vi "Page_Source_Settings_Update_Display.vi"(6 "AB_Build in":refnum<class "AB_Build.lvclass">, 8 "error in (no error)":errorcluster, 9 "ctlReferences":T3, 10 "supportedFunctions":T2, 11 "AB_Source in":refnum<class "AB_Source.lvclass">) -> (0 "error out":errorcluster, 2 "parentApplies":T1, 3 "AB_Source out":refnum<class "AB_Source.lvclass">)   [LabVIEW 2020, in "AB_Source.lvclass"]
uses:
  <vilib>/AppBuilder/AB_Classes/Source/AB_Source.lvclass
  <resource>/Framework/Providers/Builds/AppBuilder/AB_UI_Page_Source_Settings_References.ctl
  <resource>/Framework/Providers/Builds/AppBuilder/AB_UI_Page_Source_Settings_supportedFunctions.ctl
  <vilib>/AppBuilder/AB_Parent_Applies.ctl
  <vilib>/AppBuilder/AB_Classes/Build/AB_Build.lvclass
  <vilib>/AppBuilder/AB_Classes/Source/AB_Source.lvclass/AB_Source.ctl
  <vilib>/AppBuilder/AB_Source_Inclusion.ctl
  <vilib>/AppBuilder/AB_Source_Property_Type.ctl
  <resource>/Framework/Providers/Common/provcom_StringGlobals.vi
  <vilib>/AppBuilder/AB_Classes/Destination/AB_Destination.lvclass
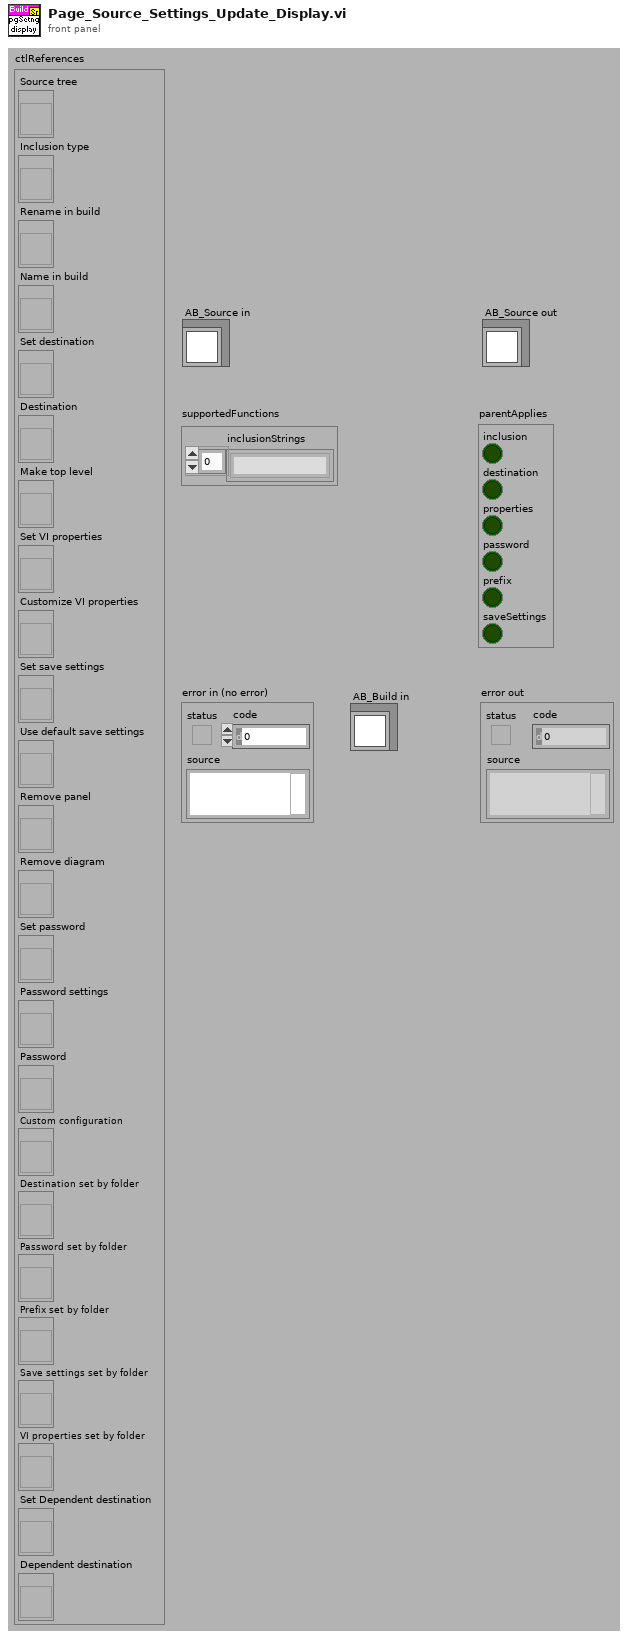
[diagram p1: front panel]
types:
  T1 = typedef "AB_Parent_Applies.ctl" = cluster{"inclusion":bool, "destination":bool, "properties":bool, "password":bool, "prefix":bool, "saveSettings":bool}
  T2 = typedef "AB_UI_Page_Source_Settings_supportedFunctions.ctl" = cluster{"inclusionStrings":string[]}
  T3 = typedef "AB_UI_Page_Source_Settings_References.ctl" = cluster{"Source tree":refnum<vi>, "Inclusion type":refnum<vi>, "Rename in build":refnum<vi>, "Name in build":refnum<vi>, "Set destination":refnum<vi>, "Destination":refnum<vi>, "Make top level":refnum<vi>, "Set VI properties":refnum<vi>, "Customize VI properties":refnum<vi>, "Set save settings":refnum<vi>, "Use default save settings":refnum<vi>, "Remove panel":refnum<vi>, "Remove diagram":refnum<vi>, "Set password":refnum<vi>, "Password settings":refnum<vi>, "Password":refnum<vi>, "Custom configuration":refnum<vi>, "Destination set by folder":refnum<vi>, "Password set by folder":refnum<vi>, "Prefix set by folder":refnum<vi>, "Save settings set by folder":refnum<vi>, "VI properties set by folder":refnum<vi>, "Set Dependent destination":refnum<vi>, "Dependent destination":refnum<vi>}
  T4 = typedef "AB_Source_Inclusion.ctl" = enum16{"IncludeIfReferenced", "Include", "Exclude", "TopLevel"}
  T5 = typedef "AB_Source_Property_Type.ctl" = enum16{"Remove block diagram", "Remove front panel", "Password", "Window has title bar", "Show menu bar", "Show vertical scroll bar", "Show horizontal scroll bar", "Show toolbar", "Show Abort button", "Show fp when called", "Window behavior", "Allow user to close window", "Window run-time position", "Run when opened", "Allow debugging", "Auto error handling", "Generate guard code", "Use stack variables", "Expression folding", "Integer only", "Inline subVI"}
  T6 = enum32{"No password change", "Remove password", "Apply new password"}
  T7 = typedef "AB_Source_Properties.ctl" = cluster{"sourcePropertyType":T5, "value":variant}
  T8 = typedef "AB_Build.ctl" = cluster{"buildSpecName":string, "buildSpecDescription":string, "destinations":refnum<class "AB_Destination.lvclass">[], "exclusionOption":T9, "defaultLanguage":string, "supportedLanguages":string[], "excludedDirectories":path[], "buildContext":refnum<vi>, "buildObject":T10, "preview":bool, "programatic":bool, "progressBarEvents":T11, "userLog_Path":path, "preActionID":string, "preAction_Path":path, "postActionID":string, "postAction_Path":path, "eng_checkForBrokenVIs?":bool, "eng_verboseLinkerErrors?":bool, "localDest_Path":path, "targetDest_Path":path, "removeVIObject":u16, "cache":refnum<class "PreviewCache.lvclass">, "use cache":bool, "previewCache_ID":string, "buildCache_ID":string, "eng_TempLocalDest_Path":path, "eng_collectDependencies?":bool, "versionInfo":cluster{"buildVersion":cluster{"major":u16, "minor":u16, "patch":u16, "build":u16}, "autoIncrement":bool}, "eng_enableVIChecksums":bool}
  T9 = typedef "AB_Exclusion_Option.ctl" = cluster{"typedefs":bool, "polymorphicVIs":bool, "unusedLibraryItems":bool, "modifyLibraryFile":bool, "edit-timeDependencies":bool, "inlineVIs":bool, "dependent PPLs":bool, "dependent DLLs":bool}
  T10 = typedef "ItemRef.ctl" = u64
  T11 = typedef "provcom_ProgressBar_Events.ctl" = cluster{"newJob":refnum<user-event>, "newItem":refnum<user-event>, "errorMsg":T12, "cancel":refnum<user-event>}
  T12 = typedef "mxLvBuildError.ctl" = refnum<user-event>
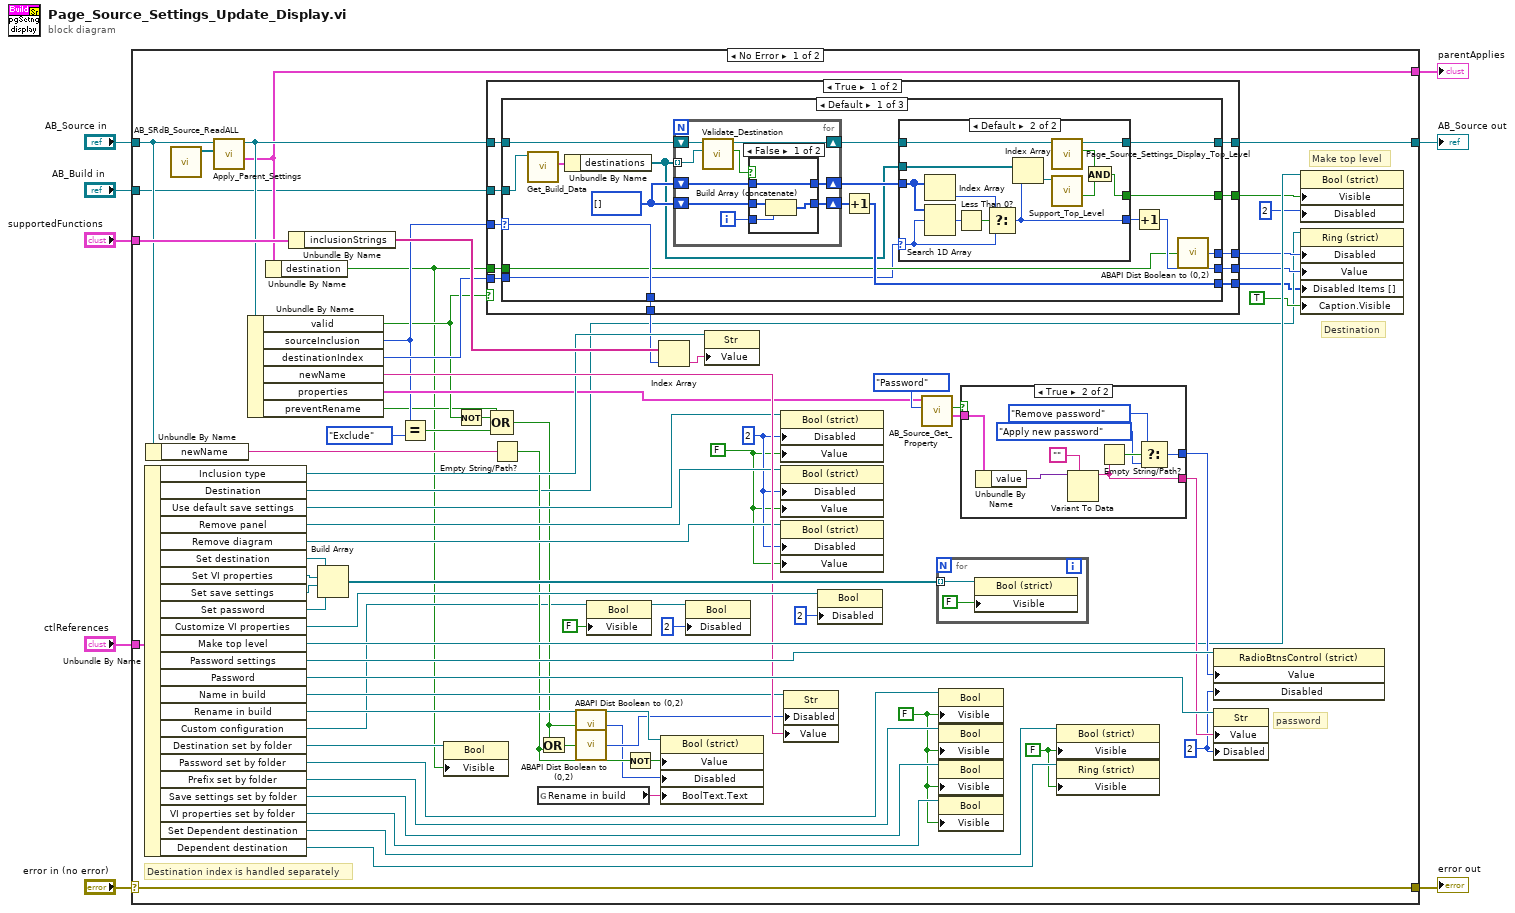
[diagram p0: block diagram]
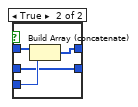
[diagram p3: hidden frame]
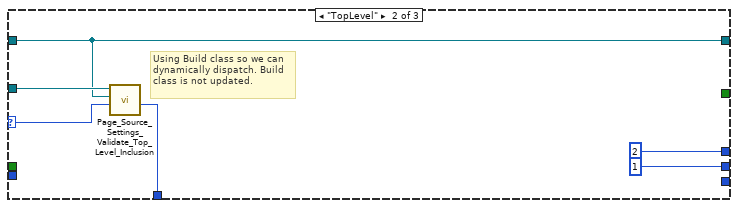
[diagram p4: hidden frame]
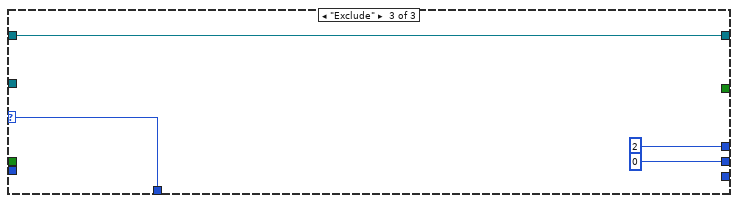
[diagram p5: hidden frame]
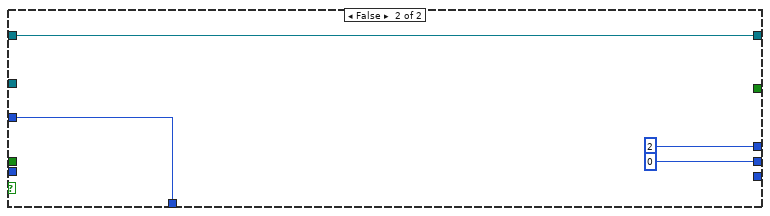
[diagram p6: hidden frame]
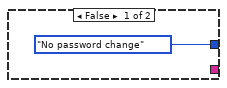
[diagram p7: hidden frame]
diagram:
  n1 = case shown="No Error" "error in (no error)" {
    selector: "error in (no error)" -> [w82 w169]
    tunnel: [w82 w169] -> w7
    tunnel: [w65 w168] -> w5
    tunnel: "AB_Source in" -> [w41 w168]
    tunnel: "ctlReferences" -> [w81 _]
    tunnel: "supportedFunctions" -> [w80 _]
    tunnel: [w58 _] -> w2
    tunnel: "AB_Build in" -> [w23 _]
    frame No Error {
      w9 = FALSE ("Visible")
      w12 = FALSE ("Visible")
      w48 = u8 2 ("Disabled")
      w47 = u8 2 ("Disabled")
      w44 = FALSE
      # "password"
      # "Make top level"
      # "Destination"
      # "Destination index is handled separately"
      n2 = Unbundle By Name(w81) -> ("Inclusion type"=w52:refnum<vi>, "Destination"=w31:refnum<vi>, "Use default save settings"=w51:refnum<vi>, "Remove panel"=w50:refnum<vi>, "Remove diagram"=w49:refnum<vi>, "Set destination"=w77:refnum<vi>, "Set VI properties"=w54:refnum<vi>, "Set save settings"=w76:refnum<vi>, "Set password"=w59:refnum<vi>, "Customize VI properties"=w74:refnum<vi>, "Make top level"=w67:refnum<vi>, "Password settings"=w73:refnum<vi>, "Password"=w71:refnum<vi>, "Name in build"=w43:refnum<vi>, "Rename in build"=w42:refnum<vi>, "Custom configuration"=w22:refnum<vi>, "Destination set by folder"=w18:refnum<vi>, "Password set by folder"=w16:refnum<vi>, "Prefix set by folder"=w15:refnum<vi>, "Save settings set by folder"=w14:refnum<vi>, "VI properties set by folder"=w13:refnum<vi>, "Set Dependent destination"=w11:refnum<vi>, "Dependent destination"=w10:refnum<vi>)
      n3 = Unbundle By Name(w41) -> ("newName"=w40:string)
      n4 = call <resource>:"AB_SRdB_Source_ReadALL.vi"() -> ("ALL data"=w46:refnum<class "AB_Source.lvclass">[])  [unwired: 10 in, 1 out]
      n5 = call-dynamic "Apply_Parent_Settings.vi"("sourceItems in"=w46, "AB_Source in"=w41) -> ("parentApplies"=w58:T1, "AB_Source out"=w68:refnum<class "AB_Source.lvclass">)  [unwired: 6 in, 2 out]
      n6 = Unbundle By Name(w68) -> ("valid"=w27:bool, "sourceInclusion"=w34:T4, "destinationIndex"=w63:i32, "newName"=w53:string, "properties"=w45:T7[], "preventRename"=w25:bool)
      n7 = Unbundle By Name(w58) -> ("destination"=w17:bool)
      n8 = Unbundle By Name(w80) -> ("inclusionStrings"=w79:string[])
      n9 = Build Array(w77, w54, w76, w59) -> (w75:refnum<vi>[])
      n10 = Equal?(x=w34, y=AB_Source_Inclusion."Exclude") -> (x = y?=w30:bool)
      n11 = property class="Bool"(reference=w18, "Visible"=w17) -> ()  [unwired: 1 in, 2 out]
      n12 = Not(x=w27) -> (.not. x?=w26:bool)
      n13 = case shown="True" w27 {
        tunnel: w68 -> [w93 w156]
        tunnel: [w92 _] -> w66
        tunnel: [w91 w156] -> w65
        tunnel: w63 -> [w90 _]
        tunnel: [w89 u8 2 ("0, 2")] -> w62
        tunnel: [w88 0] -> w61
        tunnel: [w87 _] -> w24
        tunnel: w17 -> [w84 _]
        tunnel: w34 -> [w86 w153]
        tunnel: [w85 w153] -> w32
        tunnel: w23 -> [w83 _]
        frame True {
          n14 = case shown="Default" w86 {
            selector: w86 -> [w104 w144 w149]
            tunnel: w93 -> [w110 w145 w150]
            tunnel: w90 -> [w98 _ _]
            tunnel: [w103 _ _] -> w92
            tunnel: [w96 w145 w150] -> w91
            tunnel: [w109 u8 2 ("0, 2") u8 2 ("0, 2")] -> w89
            tunnel: [w108 1 0] -> w88
            tunnel: [w107 _ _] -> w87
            tunnel: [w104 w143 w149] -> w85
            tunnel: w84 -> [w99 _ _]
            tunnel: w83 -> [w94 w146 _]
            frame Default {
              w102 = i32[] []
              n15 = call <vilib>:"Get_Build_Data.vi"("Class in"=w94) -> ("data"=w106:T8)  [unwired: 8 in, 2 out]
              n16 = Unbundle By Name(w106) -> ("destinations"=w95:refnum<class "AB_Destination.lvclass">[])
              n17 = for {
                tunnel: w95 -> [w133] mode=indexing
                shift-right: [w130] -> w100
                shift-left: w102 -> [w129]
                shift-right: [w128] -> w97
                shift-left: w110 -> [w134]
                shift-right: [w126] -> w101
                shift-left: w102 -> [w127]
                i -> [w131]
                n18 = call <vilib>:"Validate_Destination.vi"("Destination"=w133, "AB_Source in"=w134) -> ("Valid"=w132:bool, "AB_Source out"=w128:refnum<class "AB_Source.lvclass">)  [unwired: 7 in, 1 out]
                n19 = case shown="False" w132 {
                  tunnel: w131 -> [w135 w142]
                  tunnel: [w138 w141] -> w130
                  tunnel: w129 -> [w138 w140]
                  tunnel: [w136 w139] -> w126
                  tunnel: w127 -> [w137 w139]
                  frame False {
                    n20 = Build Array (concatenate)(w137, w135) -> (w136:i32[])
                  }
                  frame True {
                    n21 = Build Array (concatenate)(w140, w142) -> (w141:i32[])
                  }
                }
              }
              n22 = Increment(x=w101) -> (x+1=w107:i32[])
              n23 = case shown="Default" w98 {
                selector: w98 -> [w112 w118]
                tunnel: [w112 w123] -> w105
                tunnel: [_ w113] -> w103
                tunnel: w100 -> [_ w121]
                tunnel: w95 -> [_ w119]
                tunnel: w97 -> [w111 w117]
                tunnel: [w111 w116] -> w96
                frame -1 {
                }
                frame Default {
                  n24 = Index Array(array=w121) -> (element=w120:i32)  [unwired: 1 in]
                  n25 = Search 1D Array(1D array=w121, element=w118) -> (index of element=w124:i32)  [unwired: 1 in]
                  n26 = Less Than 0?(x=w124) -> (x < 0?=w125:bool)
                  n27 = Select(t=w120, s=w125, f=w118) -> (s? t:f=w123:i32)
                  n28 = Index Array(array=w119, index=w123) -> (element=w122:refnum<class "AB_Destination.lvclass">)
                  n29 = call-dynamic "Page_Source_Settings_Display_Top_Level.vi"("AB_Source in"=w117) -> ("displayTopLevel"=w114:bool, "AB_Source out"=w116:refnum<class "AB_Source.lvclass">)  [unwired: 8 in, 1 out]
                  n30 = call-dynamic "Support_Top_Level.vi"("AB_Destination in"=w122) -> ("displayTopLevel"=w115:bool)  [unwired: 7 in, 3 out]
                  n31 = And(x=w114, y=w115) -> (x .and. y?=w113:bool)
                }
              }
              n32 = Increment(x=w105) -> (x+1=w108:i32)
              n33 = call <vilib>:"ABAPI Dist Boolean to (0,2).vi"("Boolean"=w99) -> ("0, 2"=w109:u8)  [unwired: 4 in]
            }
            frame "TopLevel" {
              # "Using Build class so we can dynamically dispatch. Build class is not updated."
              n34 = call-dynamic "Page_Source_Settings_Validate_Top_Level_Inclusion.vi"("sourceInclusion in"=w144, "AB_Source in"=w145, "AB_Build in"=w146) -> ("sourceInclusion out"=w143:T4)  [unwired: 6 in, 2 out]
            }
            frame "Exclude" {
            }
          }
        }
        frame False {
        }
      }
      n35 = Compound Arithmetic op=OR(w25, w26, w30) -> (w29:bool)
      n36 = Empty String/Path?(string/path=w40) -> (empty?=w36:bool)
      n37 = global read "provcom_StringGlobals.vi" "Rename in build"() -> (w37:string)
      n38 = Or(x=w29, y=w36) -> (x .or. y?=w35:bool)
      n39 = call <vilib>:"ABAPI Dist Boolean to (0,2).vi"("Boolean"=w29) -> ("0, 2"=w28:u8)  [unwired: 4 in]
      n40 = call <vilib>:"ABAPI Dist Boolean to (0,2).vi"("Boolean"=w35) -> ("0, 2"=w38:u8)  [unwired: 4 in]
      n41 = property class="Bool"(reference=w22, "Visible"=FALSE) -> (reference out=w20:refnum<vi>)  [unwired: 1 in, 1 out]
      n42 = Not(x=w36) -> (.not. x?=w39:bool)
      n43 = Index Array(array=w79, index=w32) -> (element=w78:string)
      n44 = property class="Bool (strict)"(reference=w42, "Value"=w39, "Disabled"=w28, "BoolText.Text"=w37) -> ()  [unwired: 1 in, 2 out]
      n45 = property class="Bool"(reference=w20, "Disabled"=u8 2) -> ()  [unwired: 1 in, 2 out]
      n46 = property class="Str"(reference=w52, "Value"=w78) -> ()  [unwired: 1 in, 2 out]
      n47 = property class="Bool (strict)"(reference=w51, "Disabled"=w47, "Value"=w44) -> ()  [unwired: 1 in, 2 out]
      n48 = property class="Bool (strict)"(reference=w50, "Disabled"=w47, "Value"=w44) -> ()  [unwired: 1 in, 2 out]
      n49 = property class="Bool (strict)"(reference=w49, "Disabled"=w47, "Value"=w44) -> ()  [unwired: 1 in, 2 out]
      n50 = property class="Str"(reference=w43, "Disabled"=w38, "Value"=w53) -> ()  [unwired: 1 in, 2 out]
      n51 = property class="Bool"(reference=w74, "Disabled"=u8 2) -> ()  [unwired: 1 in, 2 out]
      n52 = call <vilib>:"AB_Source_Get_Property.vi"("type"=AB_Source_Property_Type."Password" ("y"), "sourceProperties in"=w45) -> ("sourceProperty"=w55:T7, "found"=w56:bool)  [unwired: 6 in, 2 out]
      n53 = for {
        tunnel: w75 -> [w166] mode=indexing
        n54 = property class="Bool (strict)"(reference=w166, "Visible"=FALSE) -> ()  [unwired: 1 in, 2 out]
      }
      n55 = property class="Bool"(reference=w16, "Visible"=w12) -> ()  [unwired: 1 in, 2 out]
      n56 = property class="Bool"(reference=w15, "Visible"=w12) -> ()  [unwired: 1 in, 2 out]
      n57 = property class="Bool"(reference=w14, "Visible"=w12) -> ()  [unwired: 1 in, 2 out]
      n58 = property class="Bool"(reference=w13, "Visible"=w12) -> ()  [unwired: 1 in, 2 out]
      n59 = case shown="True" w56 {
        tunnel: [T6."No password change" ("Value") w162] -> w72
        tunnel: [_ w160] -> w70
        tunnel: w55 -> [_ w159]
        frame False {
        }
        frame True {
          n60 = Unbundle By Name(w159) -> ("value"=w158:variant)
          n61 = Variant To Data(type="", Variant=w158) -> (data=w160:string)  [unwired: 1 in, 1 out]
          n62 = Empty String/Path?(string/path=w160) -> (empty?=w164:bool)
          n63 = Select(t=T6."Remove password" ("Value"), s=w164, f=T6."Apply new password" ("Value")) -> (s? t:f=w162:T6)
        }
      }
      n64 = property class="Bool (strict)"(reference=w11, "Visible"=w9) -> ()  [unwired: 1 in, 2 out]
      n65 = property class="Ring (strict)"(reference=w10, "Visible"=w9) -> ()  [unwired: 1 in, 2 out]
      n66 = property class="RadioBtnsControl (strict)"(reference=w73, "Value"=w72, "Disabled"=w48) -> ()  [unwired: 1 in, 2 out]
      n67 = property class="Str"(reference=w71, "Value"=w70, "Disabled"=w48) -> ()  [unwired: 1 in, 2 out]
      n68 = property class="Bool (strict)"(reference=w67, "Visible"=w66, "Disabled"=u8 2) -> ()  [unwired: 1 in, 2 out]
      n69 = property class="Ring (strict)"(reference=w31, "Disabled"=w62, "Value"=w61, "Disabled Items []"=w24, "Caption.Visible"=TRUE) -> ()  [unwired: 1 in, 2 out]
    }
    frame Error {
    }
  }
  "error out" <- w7
  "AB_Source out" <- w5
  "parentApplies" <- w2
